vi "Data Logger.vi"(8 "error in (no error)":errorcluster, 9 "Turn X joystick":dbl, 10 "Speed Y Joystick":dbl, 11 "Function":enum16{"Start Log", "Log Data", "Stop Log"}(ring)=enum."Stop Log") -> (0 "error out":errorcluster={"status"=TRUE, "code"=1430, "source"="Move in DATA LOGGER.VI->Test Data Logger.vi<APPEND>\n<Not A Path>"}, 3 "Final Filename":path)   [LabVIEW 2019]
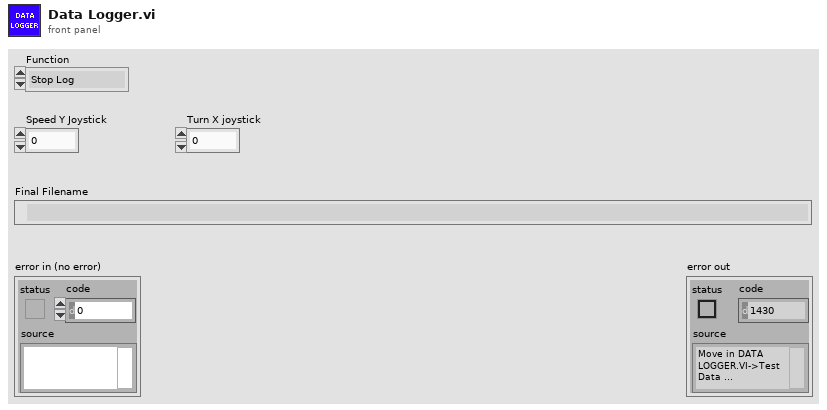
[diagram p1: front panel]
types:
  T1 = enum16{"open", "replace", "create", "open or create", "replace or create", "replace or create with confirmation"}
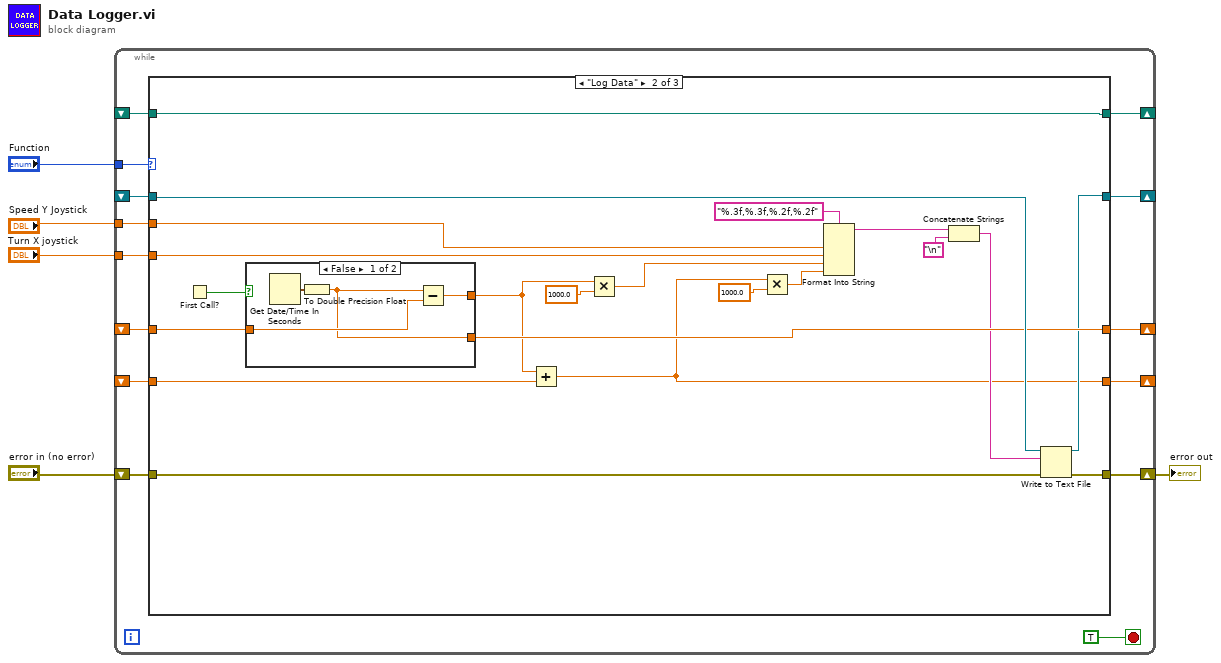
[diagram p0: block diagram]
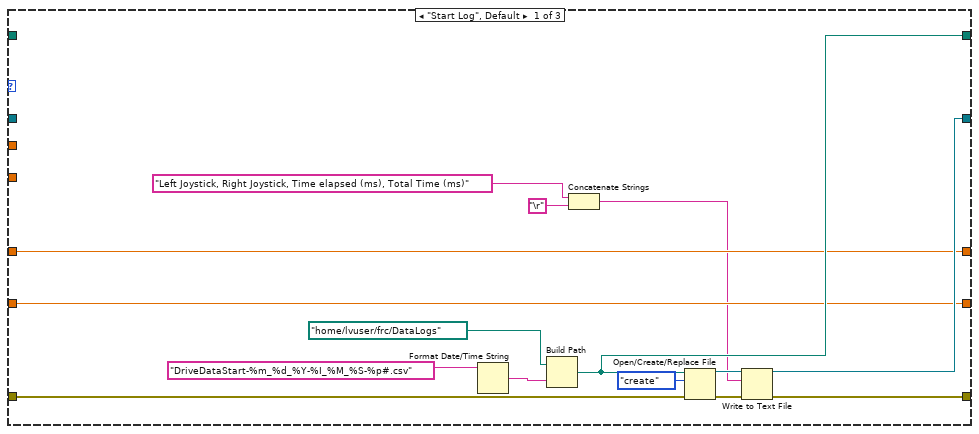
[diagram p2: hidden frame]
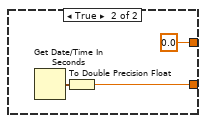
[diagram p3: hidden frame]
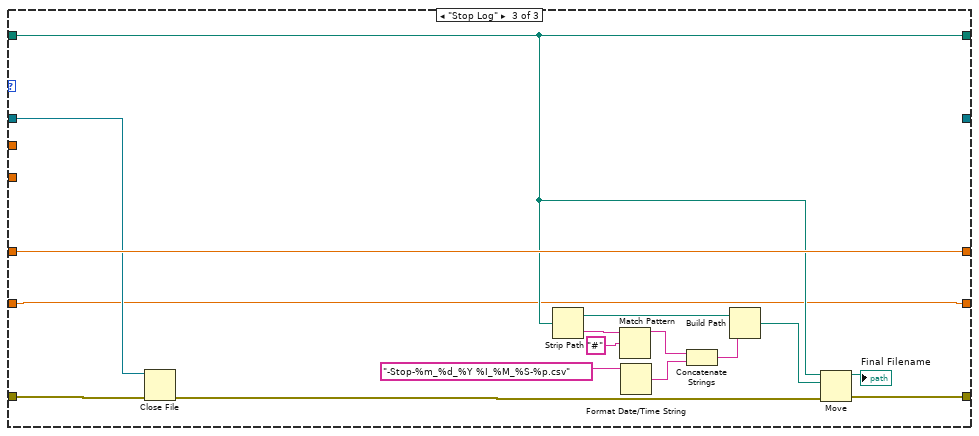
[diagram p4: hidden frame]
diagram:
  n1 = while {
    shift-right: [w18] -> w2
    shift-left: "error in (no error)" -> [w19]
    shift-right: [w17] -> _
    shift-left: _ -> [w16]
    tunnel: "Speed Y Joystick" -> [w15]
    tunnel: "Turn X joystick" -> [w14]
    tunnel: "Function" -> [w12]
    shift-right: [w11] -> _
    shift-left: _ -> [w10]
    shift-right: [w9] -> _
    shift-left: _ -> [w8]
    shift-right: [w7] -> _
    shift-left: _ -> [w6]
    stop <- TRUE stop-if-true
    n2 = case shown="\"Log Data\"" w12 {
      tunnel: [w30 w55 w70] -> w18
      tunnel: w19 -> [w32 w42 w66]
      tunnel: [w28 w52 _] -> w17
      tunnel: w16 -> [_ w54 w65]
      tunnel: w15 -> [_ w45 _]
      tunnel: w14 -> [_ w44 _]
      tunnel: [w26 w53 w68] -> w11
      tunnel: w10 -> [w26 w47 w68]
      tunnel: [w27 w51 w64] -> w9
      tunnel: w8 -> [_ w51 w64]
      tunnel: [w25 w36 w63] -> w7
      tunnel: w6 -> [w25 w40 w63]
      frame "Start Log", Default {
        n3 = Format Date/Time String(time format string (%c)="DriveDataStart-%m_%d_%Y-%I_%M_%S-%p#.csv" ("PXI Log filename format")) -> (date/time string=w34:string)  [unwired: 2 in]
        n4 = Build Path(base path=path "/home/lvuser/frc/DataLogs", name or relative path=w34) -> (appended path=w27:path)
        n5 = Concatenate Strings("Left Joystick, Right Joystick, Time elapsed (ms), Total Time (ms)" ("Column Headers"), "\r") -> (w21:string)
        n6 = Open/Create/Replace File(file path (use dialog)=w27, error in=w32, operation (0:open)=T1."create") -> (refnum out=w29:refnum<file>, error out=w31:errorcluster)  [unwired: 3 in, 1 out]
        n7 = Write to Text File(file (use dialog)=w29, text=w21, error in=w31) -> (refnum out=w28:refnum<file>, error out=w30:errorcluster)  [unwired: 1 in, 1 out]
      }
      frame "Log Data" {
        n8 = First Call?() -> (First Call?: T/F=w48:bool)
        n9 = case shown="False" w48 {
          tunnel: [w57 0.0] -> w41
          tunnel: [w56 w60] -> w53
          tunnel: w47 -> [w58 _]
          frame False {
            n10 = Get Date/Time In Seconds() -> (seconds since 1Jan1904=w59:timestamp)
            n11 = To Double Precision Float(number=w59) -> (double precision float=w56:dbl)
            n12 = Subtract(x=w56, y=w58) -> (x-y=w57:dbl)
          }
          frame True {
            n13 = Get Date/Time In Seconds() -> (seconds since 1Jan1904=w61:timestamp)
            n14 = To Double Precision Float(number=w61) -> (double precision float=w60:dbl)
          }
        }
        n15 = Add(x=w41, y=w40) -> (x+y=w36:dbl)
        n16 = Multiply(x=w41, y=1000.0) -> (x*y=w39:dbl)
        n17 = Multiply(x=w36, y=1000.0) -> (x*y=w35:dbl)
        n18 = Format Into String(format string="%.3f,%.3f,%.2f,%.2f", w45, w44, w39, w35) -> (resulting string=w43:string)  [unwired: 2 in, 1 out]
        n19 = Concatenate Strings(w43, "\n") -> (w49:string)
        n20 = Write to Text File(file (use dialog)=w54, text=w49, error in=w42) -> (refnum out=w52:refnum<file>, error out=w55:errorcluster)  [unwired: 1 in, 1 out]
      }
      frame "Stop Log" {
        n21 = Close File(refnum=w65, error in=w66) -> (error out=w67:errorcluster)  [unwired: 1 out]
        n22 = Strip Path(path=w64) -> (stripped path=w72:path, name=w74:string)
        n23 = Match Pattern(string=w74, regular expression="#") -> (before substring=w76:string)  [unwired: 1 in, 3 out]
        n24 = Format Date/Time String(time format string (%c)="-Stop-%m_%d_%Y %I_%M_%S-%p.csv") -> (date/time string=w77:string)  [unwired: 2 in]
        n25 = Concatenate Strings(w76, w77) -> (w78:string)
        n26 = Build Path(base path=w72, name or relative path=w78) -> (appended path=w73:path)
        n27 = Move(source path=w64, error in=w67, 10:w73) -> (error out=w70:errorcluster, 3:→"Final Filename":path)  [unwired: 2 in, 1 out]
      }
    }
  }
  "error out" <- w2
